vi "DIO Read.vi"(7 "DIO line":T1=1300 items=["FPGA LED"=6000, "Port3/DIO0"=1300, "Port3/DIO1"=1301, "Port3/DIO2"=1302, "Port3/DIO3"=1303, "Port3/DIO4"=1304, "Port3/DIO5"=1305, "Port3/DIO6"=1306, "Port3/DIO7"=1307, "Port3/DIO8"=1308, "Port3/DIO9"=1309], 8 "error in (no error)":errorcluster, 11 "direct IO in":refnum<class "NI_Robotics_Starter Kit Direct IO.lvclass">) -> (0 "error out":errorcluster, 2 "data":bool, 3 "direct IO out":refnum<class "NI_Robotics_Starter Kit Direct IO.lvclass">)   [LabVIEW 2017, in "NI_Robotics_Starter Kit Direct IO.lvclass"]
uses:
  <vilib>/robotics/Starter Kit/Direct IO/NI_Robotics_Starter Kit Direct IO.lvclass
  <vilib>/robotics/Starter Kit/Direct IO/DIO Lines.ctl
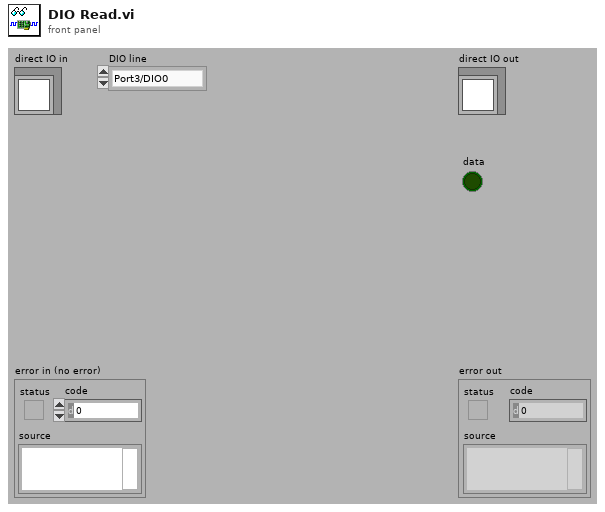
[diagram p1: front panel]
types:
  T1 = typedef "NI_Robotics_Starter Kit Direct IO.lvclass/DIO Lines.ctl" = u16
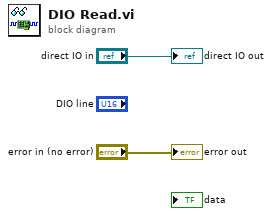
[diagram p0: block diagram]
diagram:
  "error out" <- "error in (no error)"
  "direct IO out" <- "direct IO in"
